vi "proximityCheck.vi"(5 "i":dbl, 7 "pathCoords":cluster{"x":dbl, "y":dbl}[](array[cluster]), 8 "p(t)":dbl[](array[numeric])) -> (0 "iOut":dbl, 1 "e":dbl, 2 "indexOutOfBounds":bool, 3 "p_d":dbl[](array[numeric]), 4 "WithinProximity radius":bool)   [LabVIEW 2014]
uses:
  <vilib>/imath/engines/lvmath2/RunTimeEngine/NodeEndStatement/NIMS_NodeEndStatement_Output.vi
  <instcachedir>/0/NIMS_NodeEndStatement_Output_53EC0D466D134D7ABD903AC30B43404B.lvgen/NIMS_NodeEndStatement_Output_53EC0D466D134D7ABD903AC30B43404B_001.vi
  <instcachedir>/0/NIMS_NodeEndStatement_Output_53EC0D466D134D7ABD903AC30B43404B.lvgen/NIMS_NodeEndStatement_Output_53EC0D466D134D7ABD903AC30B43404B_011.vi
  <vilib>/imath/engines/lvmath2/RunTimeEngine/ErrorHandling/NIMS_Finalize Error.vi
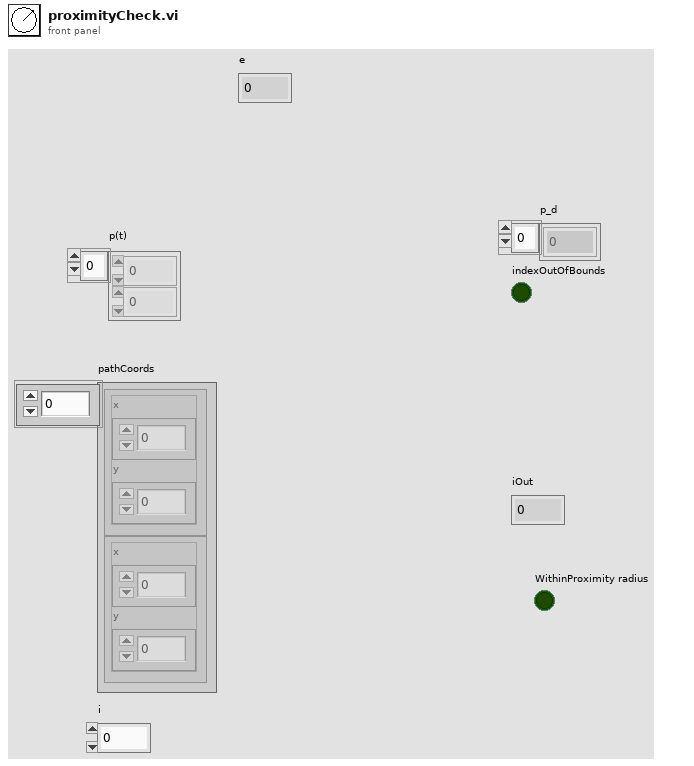
[diagram p1: front panel]
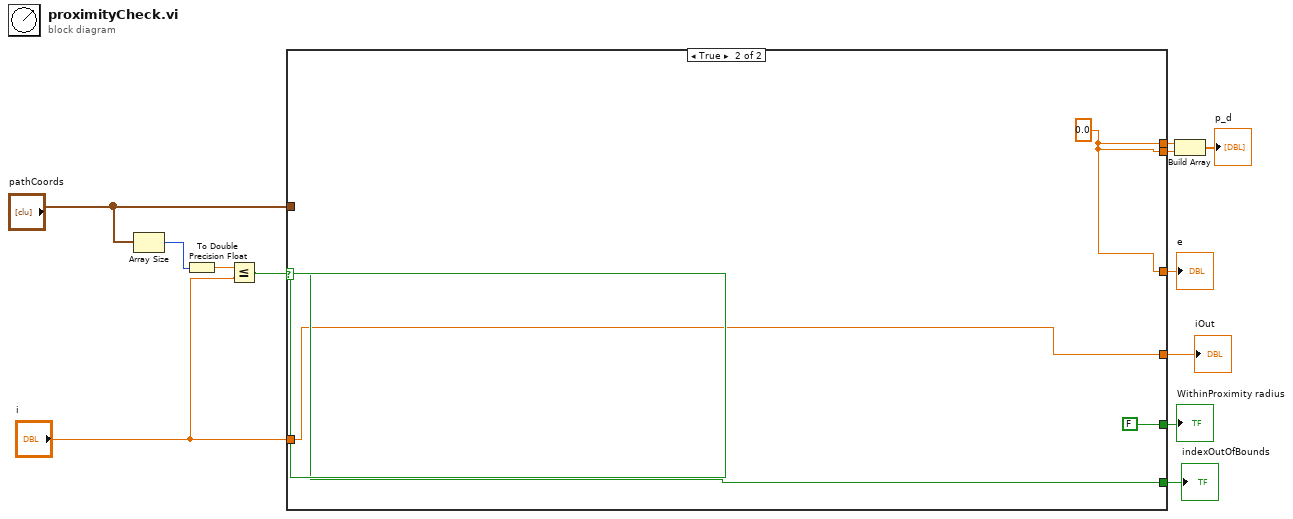
[diagram p0: block diagram]
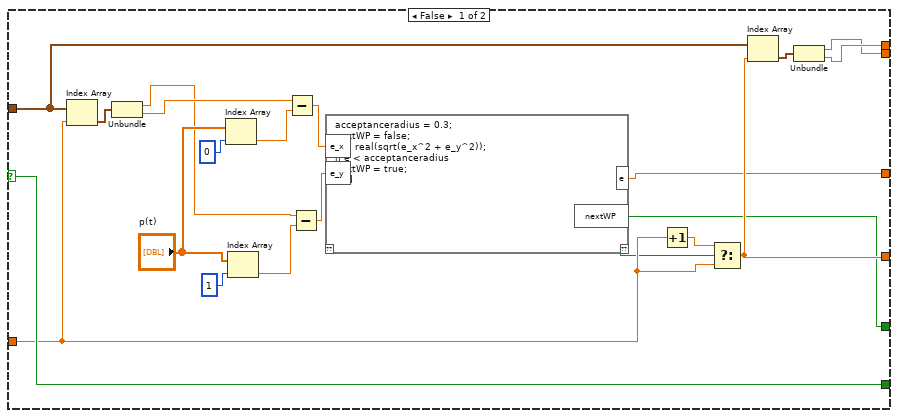
[diagram p2: hidden frame]
diagram:
  n1 = Array Size(array="pathCoords") -> (size(s)=w7:i32)
  n2 = To Double Precision Float(number=w7) -> (double precision float=w2:dbl)
  n3 = Less Or Equal?(x=w2, y="i") -> (x <= y?=w1:bool)
  n4 = case shown="True" w1 {
    selector: w1 -> [w32 w91]
    tunnel: "i" -> [w21 w88]
    tunnel: [w23 w88] -> w12
    tunnel: [w14 w90] -> w11
    tunnel: [w13 w90] -> w10
    tunnel: "pathCoords" -> [w22 _]
    tunnel: [w32 w91] -> w6
    tunnel: [w20 w90] -> w4
    tunnel: [w19 FALSE] -> w5
    frame False {
      n5 = Index Array(array=w22, index=w21) -> (element=w18:cluster{"x":dbl, "y":dbl})
      n6 = Unbundle(w18) -> ("x"=w16:dbl, "y"=w17:dbl)
      n7 = Index Array(array="p(t)", index=0) -> (element=w31:dbl)
      n8 = Index Array(array="p(t)", index=1) -> (element=w30:dbl)
      n9 = Subtract(x=w17, y=w31) -> (x-y=w24:dbl)
      n10 = Subtract(x=w16, y=w30) -> (x-y=w25:dbl)
      n11 = mathscript code="acceptanceradius = 0.3;\nnextWP = false;\ne = real(sqrt(e_x^2 + e_y^2));\nif e < acceptanceradius\nnextWP = true;\nend"("e_x"=w24, "e_y"=w25) -> ("nextWP"=w19:bool, "e"=w20:dbl)  [unwired: 1 in, 1 out]
      n12 = Increment(x=w21) -> (x+1=w26:dbl)
      n13 = Select(t=w26, s=w19, f=w21) -> (s? t:f=w23:dbl)
      n14 = Index Array(array=w22, index=w23) -> (element=w15:cluster{"x":dbl, "y":dbl})
      n15 = Unbundle(w15) -> ("x"=w13:dbl, "y"=w14:dbl)
    }
    frame True {
      w90 = 0.0
    }
  }
  "iOut" <- w12
  "indexOutOfBounds" <- w6
  "WithinProximity radius" <- w5
  "e" <- w4
  n16 = Build Array(w11, w10) -> (→"p_d":dbl[])
